vi "Toolkit - Cluster Control.vi"() -> ()   [LabVIEW 2017]
doc: "Alphabetizes a cluster control using VI scripting and the ACE toolkit VIs"
uses:
  <vilib>/Utility/traverseref.llb/TRef TravTarget.ctl
  <vilib>/Utility/traverseref.llb/VI Scripting - Traverse.lvlib
  Toolkit/Toolkit.lvlib
panel:
  out "Change?":bool
  # "Overview: Demonstrates alphabetizing a cluster control using VI scripting the ACE toolkit\nInstructions:\n1. Run this VI"
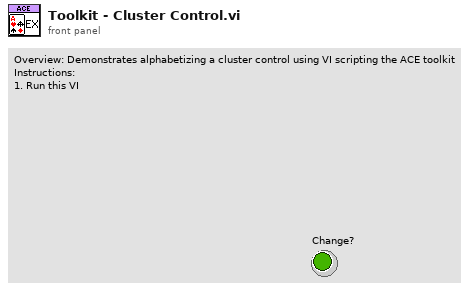
[diagram p1: front panel]
types:
  T1 = enum32{"Invalid", "Standard", "Closed", "Hidden", "Minimized", "Maximized"}
  T2 = typedef "TRef TravTarget.ctl" = enum16{"FP", "BD", "Other"}
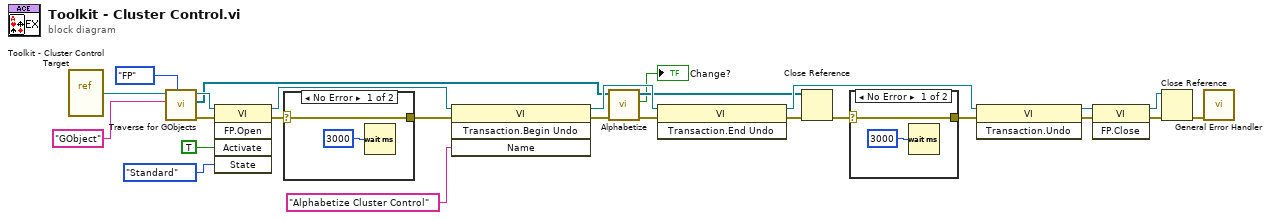
[diagram p0: block diagram]
diagram:
  n1 = vi-ref "Toolkit - Cluster Control Target.vi"() -> (w1:refnum<vi>)
  n2 = call <vilib>:"Traverse for GObjects.vi"("Traverse Target"=TRef_TravTarget."FP", "Class Name"="GObject", "VI Refnum"=w1) -> ("error out"=w21:errorcluster, "References"=w6:refnum<vi>[], "dup VI Refnum"=w20:refnum<vi>)  [unwired: 5 in, 1 out]
  n3 = invoke class="VI" method="FP.Open"(reference=w20, error in=w21, "Activate"=TRUE ("Activate?"), "State"=T1."Standard") -> (reference out=w19:refnum<vi>, error out=w18:errorcluster)  [unwired: 1 in, 3 out]
  n4 = case shown="No Error" w18 {
    selector: w18 -> [w28 w29]
    tunnel: [w28 w29] -> w15
    frame No Error {
      n5 = Wait (ms)(milliseconds to wait=u32 3000) -> ()  [unwired: 1 out]
    }
    frame Error {
    }
  }
  n6 = invoke class="VI" method="Transaction.Begin Undo"(reference=w19, error in=w15, "Name"="Alphabetize Cluster Control") -> (reference out=w13:refnum<vi>, error out=w2:errorcluster)  [unwired: 1 in, 2 out]
  n7 = call "Alphabetize.vi"("Error In"=w2, "Clusters In"=w6) -> ("Error Out"=w3:errorcluster, "Change?"=→"Change?":bool, "Clusters Out"=w5:refnum<vi>[])  [unwired: 7 in]
  n8 = invoke class="VI" method="Transaction.End Undo"(reference=w13, error in=w3) -> (reference out=w11:refnum<vi>, error out=w12:errorcluster)  [unwired: 1 in, 1 out]
  n9 = Close Reference(reference=w5, error in (no error)=w12) -> (error out=w17:errorcluster)
  n10 = case shown="No Error" w17 {
    selector: w17 -> [w31 w32]
    tunnel: [w31 w32] -> w16
    frame No Error {
      n11 = Wait (ms)(milliseconds to wait=u32 3000) -> ()  [unwired: 1 out]
    }
    frame Error {
    }
  }
  n12 = invoke class="VI" method="Transaction.Undo"(reference=w11, error in=w16) -> (reference out=w10:refnum<vi>, error out=w9:errorcluster)  [unwired: 1 in, 1 out]
  n13 = invoke class="VI" method="FP.Close"(reference=w10, error in=w9) -> (reference out=w8:refnum<vi>, error out=w7:errorcluster)  [unwired: 1 in, 1 out]
  n14 = Close Reference(reference=w8, error in (no error)=w7) -> (error out=w24:errorcluster)
  n15 = call <vilib>:"General Error Handler.vi"("error in (no error)"=w24) -> ()  [unwired: 10 in, 5 out]
